vi "Can Script Property Accessor.vi"(8 "error in (no error)":errorcluster, 11 "BaseAccessorScripter in":refnum<class "BaseAccessorScripter.lvclass">) -> (0 "error out":errorcluster, 2 "Can Script Property Accessor":bool=TRUE, 3 "BaseAccessorScripter out":refnum<class "BaseAccessorScripter.lvclass">)   [LabVIEW 2021, in "MemberVICreation.lvlib" / "BaseAccessorScripter.lvclass"]
doc: "Returns whether or not this scripter can create a valid property accessor. Array scripters cannot do this"
uses:
  <resource>/Framework/Providers/LVClassLibrary/NewAccessors/BaseAccessorScripter/BaseAccessorScripter.lvclass
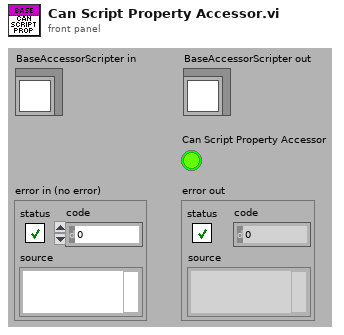
[diagram p1: front panel]
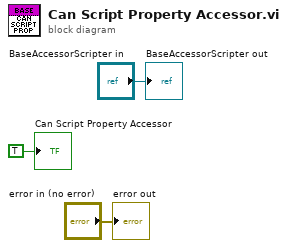
[diagram p0: block diagram]
diagram:
  "error out" <- "error in (no error)"
  "BaseAccessorScripter out" <- "BaseAccessorScripter in"
  "Can Script Property Accessor" <- TRUE ("Can Script Property Accessor")
